vi "clear_usb_buffer.vi"(0 "reference (in)":i32, 5 "error in (no error)":errorcluster, 7 "dialog? (T)":bool=TRUE) -> (14 "reference (out)":i32, 19 "error out":errorcluster)   [LabVIEW 2020, in "classes.lvlib" / "_Controller.lvclass"]
doc: "Clears the buffer on the PC as well as the USB controller. \n\nImplementss the USB Communication API function \"fnPerformaxComFlush\".\n\nProduced By:\n\n<B>Kod Integrations, LLC</B>\n4835 Marianne Drive\nMount Airy, MD 21771\nhttp://www.kodintegrations.com\nemail: info@kodintegrations.com\nphone: (240) 687-1288"
uses:
  classes/Controller/_Controller.lvclass
  Program Files (x86)/Arcus Technology/Drivers, Libraries, Source/Performax USB v4.01/PerformaxCom.dll
  libraries/common.lvlib
  common/controls/error_actions.ctl
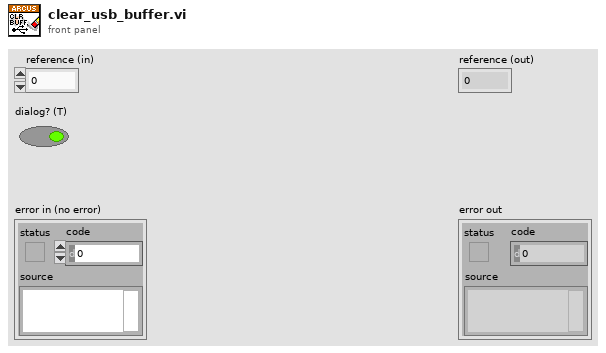
[diagram p1: front panel]
types:
  T1 = typedef "common.lvlib/error_actions.ctl" = enum16{"clearBuff", "closeRef", "nodeErr", "noDeviceInfo", "noDevices", "openRef", "sendReceive", "setTimeouts", "unknown"}
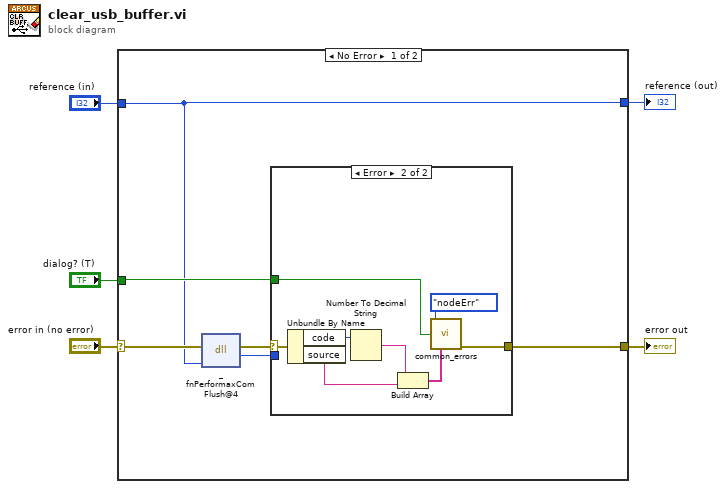
[diagram p0: block diagram]
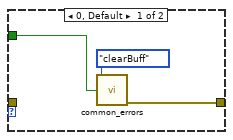
[diagram p3: hidden frame]
diagram:
  n1 = case shown="No Error" "error in (no error)" {
    selector: "error in (no error)" -> [w8 w29]
    tunnel: [w7 w29] -> w4
    tunnel: "reference (in)" -> [w6 w28]
    tunnel: [w6 w28] -> w2
    tunnel: "dialog? (T)" -> [w9 _]
    frame No Error {
      n2 = dll-call lib="C:/Program Files (x86)/Arcus Technology/Drivers, Libraries, Source/Performax USB v4.01/PerformaxCom.dll" fn="_fnPerformaxComFlush@4"(error in=w8, "reference"=w6) -> (error out=w11:errorcluster, "success"=w10:i32)  [unwired: 3 in, 1 out]
      n3 = case shown="Error" w11 {
        selector: w11 -> [w12 w24]
        tunnel: [w15 w27] -> w7
        tunnel: w10 -> [w14 _]
        tunnel: w9 -> [w13 w26]
        frame No Error {
          n4 = case shown="1" w14 {
            tunnel: [w17 w19] -> w15
            tunnel: w12 -> [_ w19]
            tunnel: w13 -> [w16 _]
            frame 0, Default {
              n5 = call "common_errors.vi"("common_errors"=error_actions."clearBuff" ("errors"), "dialog? (T)"=w16) -> ("error out"=w17:errorcluster)  [unwired: 13 in]
            }
            frame 1 {
              # "Command Successful!"
            }
          }
        }
        frame Error {
          n6 = Unbundle By Name(w24) -> ("code"=w23:i32, "source"=w21:string)
          n7 = Number To Decimal String(number=w23) -> (decimal integer string=w22:string)  [unwired: 1 in]
          n8 = Build Array(w22, w21) -> (w20:string[])
          n9 = call "common_errors.vi"("common_errors"=error_actions."nodeErr" ("errors"), "dialog? (T)"=w26, "supp_text"=w20) -> ("error out"=w27:errorcluster)  [unwired: 12 in]
        }
      }
    }
    frame Error {
    }
  }
  "error out" <- w4
  "reference (out)" <- w2
